vi "Position FIFO.vi"(11 "Loop Iteration":i32) -> (3 "Point":T1)   [LabVIEW 2014, in "Initialization and IO Node Scripting.lvlib"]
uses:
  Initialization and IO Node Scripting.lvlib
  <vilib>/XNodeSupport/XNodePoint.ctl
  <vilib>/XNodeSupport/XNodeInt.ctl
  <vilib>/XNodeSupport/NI_XNodeSupport.lvlib
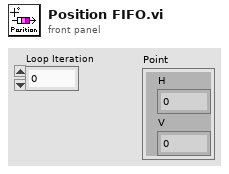
[diagram p1: front panel]
types:
  T1 = typedef "NI_XNodeSupport.lvlib/XNodePoint.ctl" = cluster{"H":T2, "V":T2}
  T2 = typedef "NI_XNodeSupport.lvlib/XNodeInt.ctl" = i32
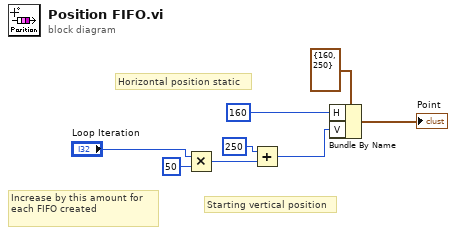
[diagram p0: block diagram]
diagram:
  # "Increase by this amount for each FIFO created"
  # "Starting vertical position"
  # "Horizontal position static"
  n1 = Multiply(x="Loop Iteration", y=50) -> (x*y=w6:i32)
  n2 = Add(x=250, y=w6) -> (x+y=w8:i32)
  n3 = Bundle By Name(cluster=T1 {"H"=160, "V"=250} ("Point"), "H"=160, "V"=w8) -> (→"Point":T1)
